vi "New Logging Thread.vi"(5 "FIFO Options":T2, 7 "fifo depths (100)":u32=100, 8 "error in (no error)":errorcluster, 10 "thread settings":T1={"Priority"=100, "Processor"=-2}, 11 "log file directory":path) -> (0 "error out":errorcluster, 2 "Logging Interface":refnum<class "Logging Interface.lvclass">, 3 "Logging Thread out":refnum<class "Logging Thread.lvclass">)   [LabVIEW 2017, in "DSF Core.lvlib" / "Logging Thread.lvclass"]
uses:
  Logging Thread.lvclass
  C:/Git/DSF/Core/Classes/Thread/Thread.lvclass
  Typedefs/DSF FIFO Options.ctl
  Interface/Logging/Logging Interface.lvclass
  Thread Settings.ctl
  Logging Thread.lvclass/Logging Thread.ctl
  Thread.lvclass
  Framework/Framework.lvclass
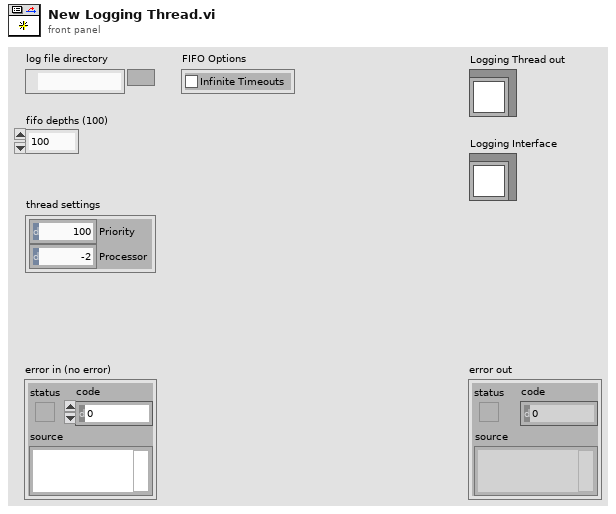
[diagram p1: front panel]
types:
  T1 = typedef "DSF Core.lvlib/Thread.lvclass/Thread Settings.ctl" = cluster{"Priority":u16, "Processor":i32}
  T2 = typedef "DSF Core.lvlib/Framework.lvclass/DSF FIFO Options.ctl" = cluster{"Infinite Timeouts":bool}
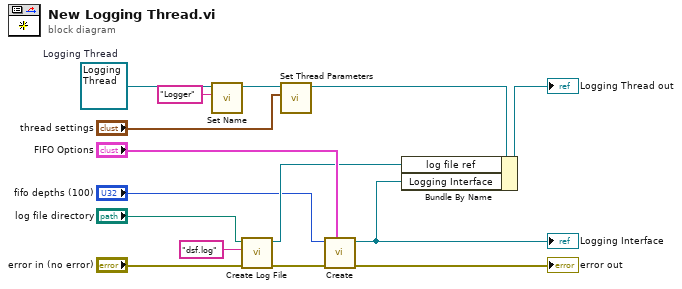
[diagram p0: block diagram]
diagram:
  w6 = refnum<class "Logging Thread.lvclass"> refnum  # Logging Thread
  n1 = call "Set Name.vi"("name"="Logger", "Thread in"=w6) -> ("Thread out"=w5:refnum<class "Logging Thread.lvclass">)  [unwired: 9 in]
  n2 = call "Create Log File.vi"("error in (no error)"="error in (no error)", "log file name"="dsf.log" ("name or relative path"), "log file directory"="log file directory") -> ("error out"=w11:errorcluster, "file refnum"=w8:refnum<file>)  [unwired: 7 in]
  n3 = call "Set Thread Parameters.vi"("thread settings"="thread settings", "Thread in"=w5) -> ("Thread out"=w4:refnum<class "Logging Thread.lvclass">)  [unwired: 9 in]
  n4 = call "Create.vi"("FIFO Options"="FIFO Options", "error in (no error)"=w11, "fifo/queue depths (10)"="fifo depths (100)") -> ("error out"=→"error out":errorcluster, "Logging Interface out"=w3:refnum<class "Logging Interface.lvclass">)  [unwired: 7 in]
  "Logging Interface" <- w3
  n5 = Bundle By Name(cluster=w4, "log file ref"=w8, "Logging Interface"=w3) -> (→"Logging Thread out":refnum<class "Logging Thread.lvclass">)
